vi "Compare_Logs.vi"() -> ()   [LabVIEW 2022 SP3]
panel:
  out "Answer":dbl
  in  "Natural log":bool
  in  "Number":dbl
  # "Compare_Logs:\nTo calculate either the natural log\nof a number, or log base-10 of a \nnumber, enter the number, and \nselect the operation using the switch."
  # "Base 10"
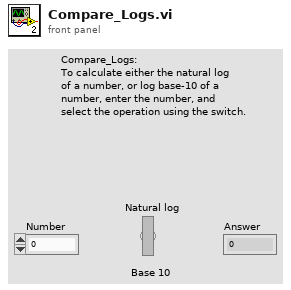
[diagram p1: front panel]
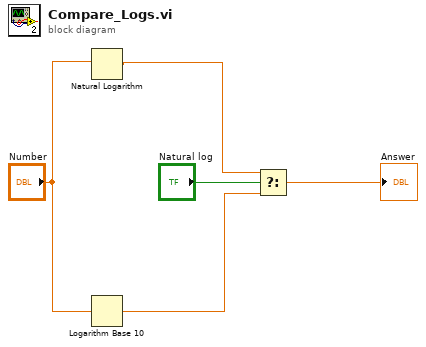
[diagram p0: block diagram]
diagram:
  n1 = Natural Logarithm(1:"Number") -> (0:w3:dbl)
  n2 = Logarithm Base 10(1:"Number") -> (0:w2:dbl)
  n3 = Select(t=w3, s="Natural log", f=w2) -> (s? t:f=→"Answer":dbl)
